vi "GetObjectName.vi"(6 "error in":errorcluster, 9 "GObject in":refnum<class "GObject.lvclass">) -> (0 "error out":errorcluster, 3 "GObject out":refnum<class "GObject.lvclass">, 4 "Name":string)   [LabVIEW 2014, in "GObject.lvclass"]
uses:
  GObject.lvclass
  Generic/Generic.lvclass/Generic.ctl
  Generic/Generic.lvclass
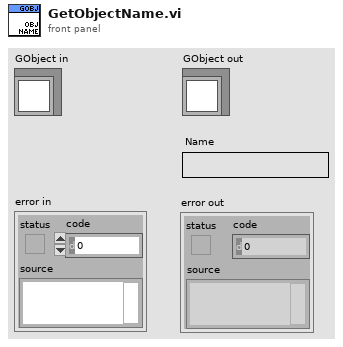
[diagram p1: front panel]
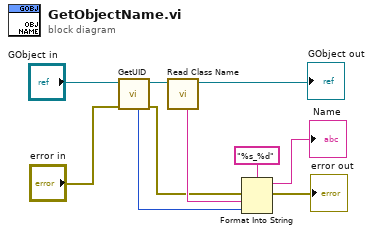
[diagram p0: block diagram]
diagram:
  n1 = call-dynamic "GetUID.vi"("error in"="error in", "GObject in"="GObject in") -> ("error out"=w1:errorcluster, "GObject out"=w6:refnum<class "GObject.lvclass">, "UID"=w9:i32)  [unwired: 5 in]
  n2 = call "Read Class Name.vi"("Generic in"=w6) -> ("Generic out"=→"GObject out":refnum<class "GObject.lvclass">, "Class Name"=w10:string)  [unwired: 7 in]
  n3 = Format Into String(format string="%s_%d", error in=w1, w10, w9) -> (resulting string=→"Name":string, error out=→"error out":errorcluster)  [unwired: 1 in]
